vi "PantherLAB_Log - Create New DQMH Event.vi"(9 "Ephemeral Scripting Info":T1, 10 "Event Info":T2 {"timeout (ms)" min=-1 step=1}, 11 "Module Info":T5) -> (0 "error out":errorcluster)   [LabVIEW 2016]
doc: "_____\nCreated using DQMH Framework: Event Scripter 7.1.0.1450."
uses:
  <vilib>/Delacor/Delacor QMH/Libraries/_Scripting Support/Module Info--cluster.ctl
  <vilib>/Delacor/Delacor QMH/Libraries/_Scripting Support/Module Type--enum.ctl
  <vilib>/Delacor/Delacor QMH/Libraries/_Scripting Support/Event Info (New)--cluster.ctl
  <vilib>/Delacor/Delacor QMH/Libraries/_Scripting Support/Event Type (New)--enum.ctl
  <vilib>/Delacor/Delacor QMH/Libraries/_Scripting Support/Request Scoping--enum.ctl
  <vilib>/Delacor/Delacor QMH/Libraries/_Scripting Support/Ephemeral Scripting Info--cluster.ctl
  PantherDashboard Scripting Hooks/PantherLAB_Log.lvlib
  <vilib>/Delacor/Delacor QMH/Libraries/_Scripting Support/dqmh_lib_DQMH Scripting Support.lvlib
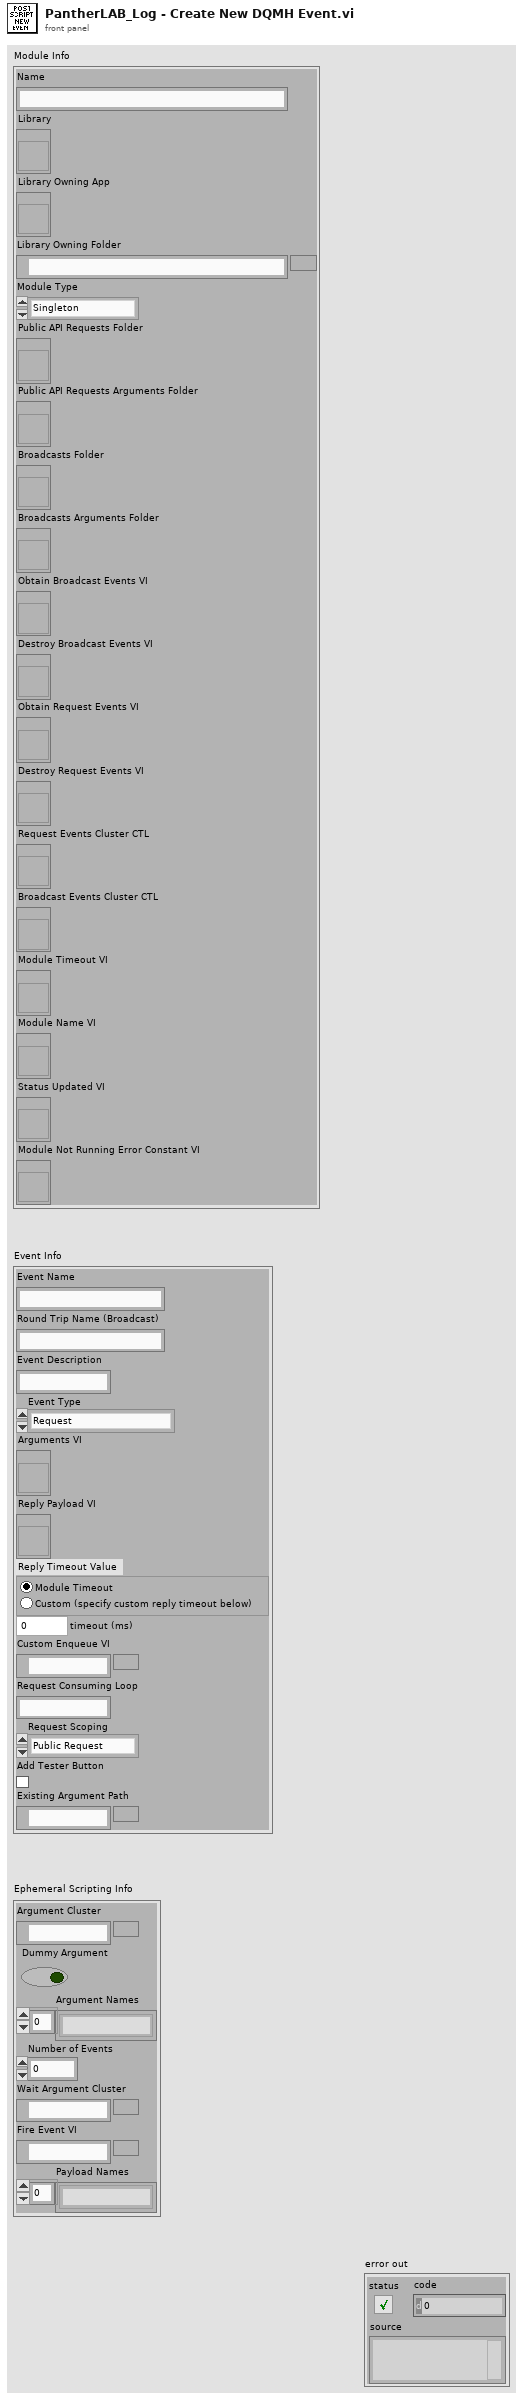
[diagram p1: front panel]
types:
  T1 = typedef "dqmh_lib_DQMH Scripting Support.lvlib/Ephemeral Scripting Info--cluster.ctl" = cluster{"Argument Cluster":path, "Dummy Argument":bool, "Argument Names":string[], "Number of Events":i32, "Wait Argument Cluster":path, "Fire Event VI":path, "Payload Names":string[]}
  T2 = typedef "dqmh_lib_DQMH Scripting Support.lvlib/Event Info (New)--cluster.ctl" = cluster{"Event Name":string, "Round Trip Name (Broadcast)":string, "Event Description":string, "Event Type":T3, "Arguments VI":refnum<vi>, "Reply Payload VI":refnum<vi>, "Reply Timeout Value":enum32{"Module Timeout", "Custom"}, "timeout (ms)":i32, "Custom Enqueue VI":path, "Request Consuming Loop":string, "Request Scoping":T4, "Add Tester Button":bool, "Existing Argument Path":path}
  T3 = typedef "dqmh_lib_DQMH Scripting Support.lvlib/Event Type (New)--enum.ctl" = enum16{"Request", "Broadcast", "Request and Wait for Reply", "Round Trip"}
  T4 = typedef "dqmh_lib_DQMH Scripting Support.lvlib/Request Scoping--enum.ctl" = enum16{"Public Request", "Private Request", "Local Instance"}
  T5 = typedef "dqmh_lib_DQMH Scripting Support.lvlib/Module Info--cluster.ctl" = cluster{"Name":string, "Library":refnum<vi>, "Library Owning App":refnum<vi>, "Library Owning Folder":path, "Module Type":T6, "Public API Requests Folder":refnum<vi>, "Public API Requests Arguments Folder":refnum<vi>, "Broadcasts Folder":refnum<vi>, "Broadcasts Arguments Folder":refnum<vi>, "Obtain Broadcast Events VI":refnum<vi>, "Destroy Broadcast Events VI":refnum<vi>, "Obtain Request Events VI":refnum<vi>, "Destroy Request Events VI":refnum<vi>, "Request Events Cluster CTL":refnum<vi>, "Broadcast Events Cluster CTL":refnum<vi>, "Module Timeout VI":refnum<vi>, "Module Name VI":refnum<vi>, "Status Updated VI":refnum<vi>, "Module Not Running Error Constant VI":refnum<vi>}
  T6 = typedef "dqmh_lib_DQMH Scripting Support.lvlib/Module Type--enum.ctl" = enum16{"Singleton", "Cloneable"}
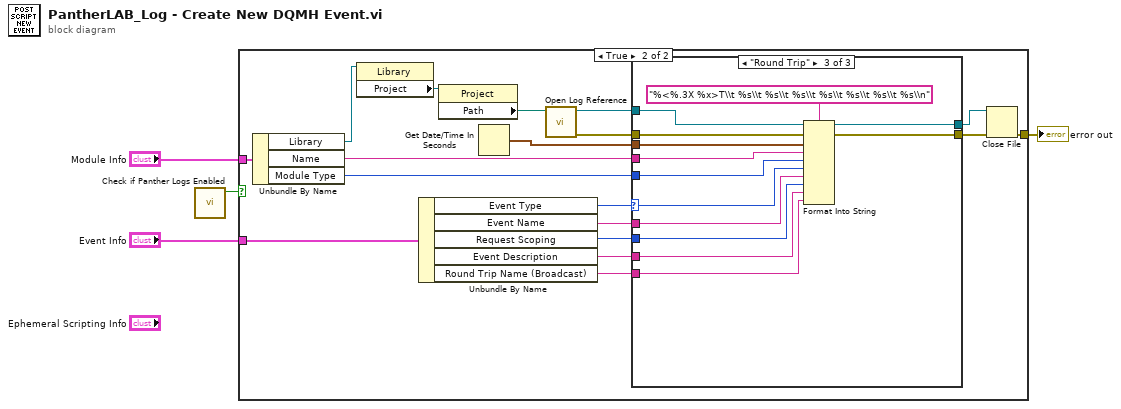
[diagram p0: block diagram]
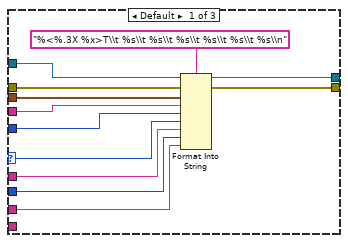
[diagram p3: hidden frame]
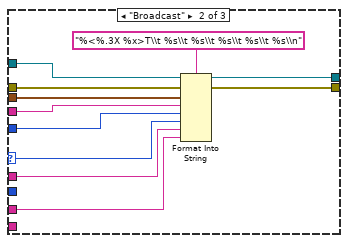
[diagram p4: hidden frame]
diagram:
  n1 = call "Check if Panther Logs Enabled.vi"() -> ("PantherLogs Enabled?"=w1:bool)  [unwired: 11 in]
  n2 = case shown="True" w1 {
    tunnel: [_ w20] -> w4
    tunnel: "Module Info" -> [_ w19]
    tunnel: "Event Info" -> [_ w16]
    frame False {
    }
    frame True {
      n3 = Unbundle By Name(w19) -> ("Library"=w18:refnum<vi>, "Name"=w8:string, "Module Type"=w7:T6)
      n4 = property class="Library"(reference=w18) -> ("Project"=w17:refnum<vi>)  [unwired: 1 in, 2 out]
      n5 = Unbundle By Name(w16) -> ("Event Type"=w14:T3, "Event Name"=w12:string, "Request Scoping"=w11:T4, "Event Description"=w10:string, "Round Trip Name (Broadcast)"=w9:string)
      n6 = property class="Project"(reference=w17) -> ("Path"=w5:path)  [unwired: 1 in, 2 out]
      n7 = Get Date/Time In Seconds() -> (seconds since 1Jan1904=w6:timestamp)
      n8 = call "Open Log Reference.vi"("Project Path"=w5) -> ("error out"=w22:errorcluster, "File Reference"=w15:refnum<file>)  [unwired: 9 in]
      n9 = case shown="\"Round Trip\"" w14 {
        selector: w14 -> [w30 w41 w54]
        tunnel: w15 -> [w32 w43 w56]
        tunnel: w22 -> [w34 w45 w58]
        tunnel: [w31 w42 w55] -> w13
        tunnel: [w33 w44 w57] -> w21
        tunnel: w12 -> [w29 w40 w53]
        tunnel: w11 -> [w28 _ w52]
        tunnel: w10 -> [w27 w39 w51]
        tunnel: w9 -> [_ _ w50]
        tunnel: w8 -> [w25 w37 w48]
        tunnel: w7 -> [w26 w38 w49]
        tunnel: w6 -> [w24 w36 w47]
        frame Default {
          n10 = Format Into String(format string="%<%.3X %x>T\\t %s\\t %s\\t %s\\t %s\\t %s\\t %s\\n", initial string=w32, error in=w34, w24, w25, w26, w30, w29, w28, w27) -> (resulting string=w31:refnum<file>, error out=w33:errorcluster)
        }
        frame "Broadcast" {
          n11 = Format Into String(format string="%<%.3X %x>T\\t %s\\t %s\\t %s\\t %s\\t %s\\n", initial string=w43, error in=w45, w36, w37, w38, w41, w40, w39) -> (resulting string=w42:refnum<file>, error out=w44:errorcluster)
        }
        frame "Round Trip" {
          n12 = Format Into String(format string="%<%.3X %x>T\\t %s\\t %s\\t %s\\t %s\\t %s\\t %s\\t %s\\n", initial string=w56, error in=w58, w47, w48, w49, w54, w53, w52, w51, w50) -> (resulting string=w55:refnum<file>, error out=w57:errorcluster)
        }
      }
      n13 = Close File(refnum=w13, error in=w21) -> (error out=w20:errorcluster)  [unwired: 1 out]
    }
  }
  "error out" <- w4
